vi "blackman_window_2.vi"() -> ()   [LabVIEW 2021]
uses:
  <vilib>/Analysis/4window.llb/Blackman-Harris Window (DBL).vi
  <vilib>/Analysis/4window.llb/AllCosWindow (DBL).vi
  <vilib>/Analysis/NI_AALPro.lvlib
panel:
  out "Init Data Out":fxp<+,16,0>[](array[numeric])
  out "Waveform Graph":dbl[](graph)
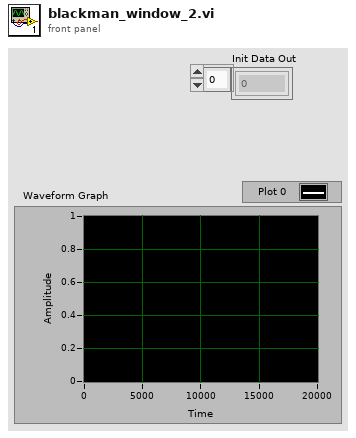
[diagram p1: front panel]
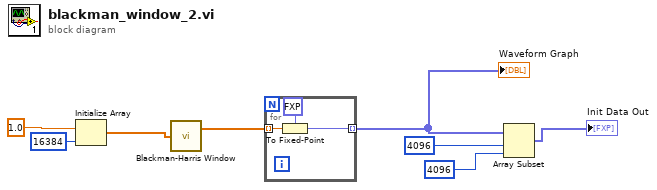
[diagram p0: block diagram]
diagram:
  n1 = Initialize Array(1.0 ("element"), 16384 ("dimension size")) -> (w6:dbl[])
  n2 = call-poly <vilib>:"Blackman-Harris Window.vi"("X"=w6) -> ("Windowed X"=w5:dbl[])  [unwired: 1 out]
  n3 = for {
    tunnel: w5 -> [w11] mode=indexing
    tunnel: [w10] -> w4 mode=indexing
    n4 = To Fixed-Point(fixed-point type=fxp<+,16,0> 0.0, number=w11) -> (fixed-point=w10:fxp<+,16,0>)
  }
  "Waveform Graph" <- w4
  n5 = Array Subset(array=w4, index=4096, length=4096) -> (→"Init Data Out":fxp<+,16,0>[])
